vi "2086查询波浪仪参数.vi"(8 "error in (no error)":errorcluster, 10 "database":string="database1.mdb", 11 "table":string) -> (0 "error out":errorcluster, 1 "database溢出":bool, 2 "有数据":bool, 3 "data":string[][](array[string]), 4 "拆分数据":bool, 5 "columns":string[](array[string]))   [LabVIEW 2016, in "数据传输系统-05.lvlib"]
uses:
  <vilib>/Utility/sysdir.llb/System Directory Type.ctl
  <vilib>/addons/database/Connection.llb/DB Tools Open Connec (String).vi
  <vilib>/addons/database/Connection.llb/Conn Execute.vi
  <vilib>/addons/database/Recordset.llb/Rec Fetch Recordset Data (R).vi
  <vilib>/addons/database/Recordset.llb/Rec Destroy - Connection.vi
  <vilib>/addons/database/_DB Variant To Data/Database Variant To Data.xnode
  <vilib>/addons/database/NI_Database_API.lvlib
panel:
  out "连接的字符串":string
  out "结果字符串":string
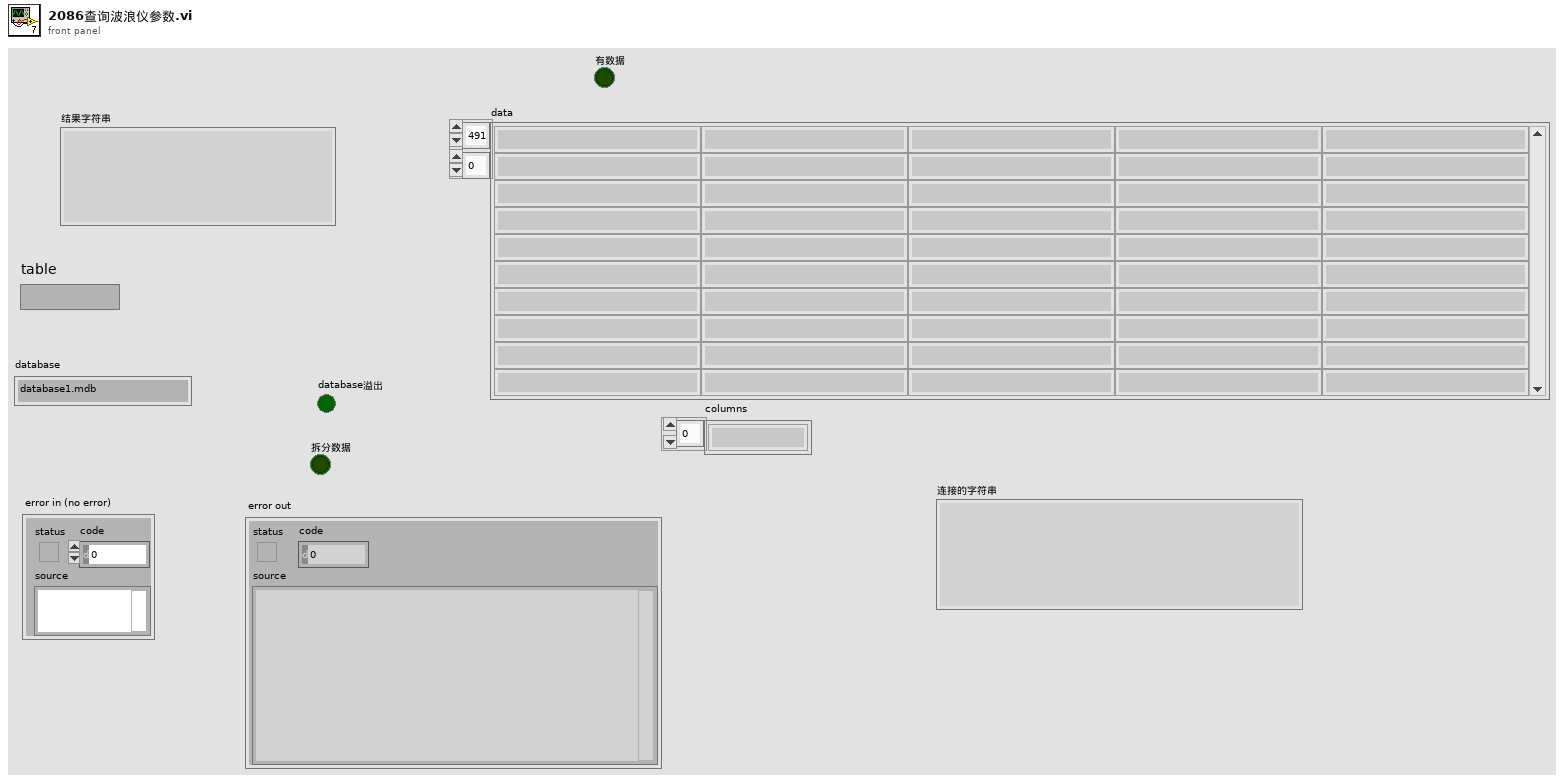
[diagram p1: front panel]
types:
  T1 = typedef "System Directory Type.ctl" = i32
  T2 = typedef "NI_Database_API.lvlib/Conn ObjectReference.ctl" = refnum<k1>
  T3 = typedef "NI_Database_API.lvlib/Rec ObjectReference.ctl" = refnum<k1>
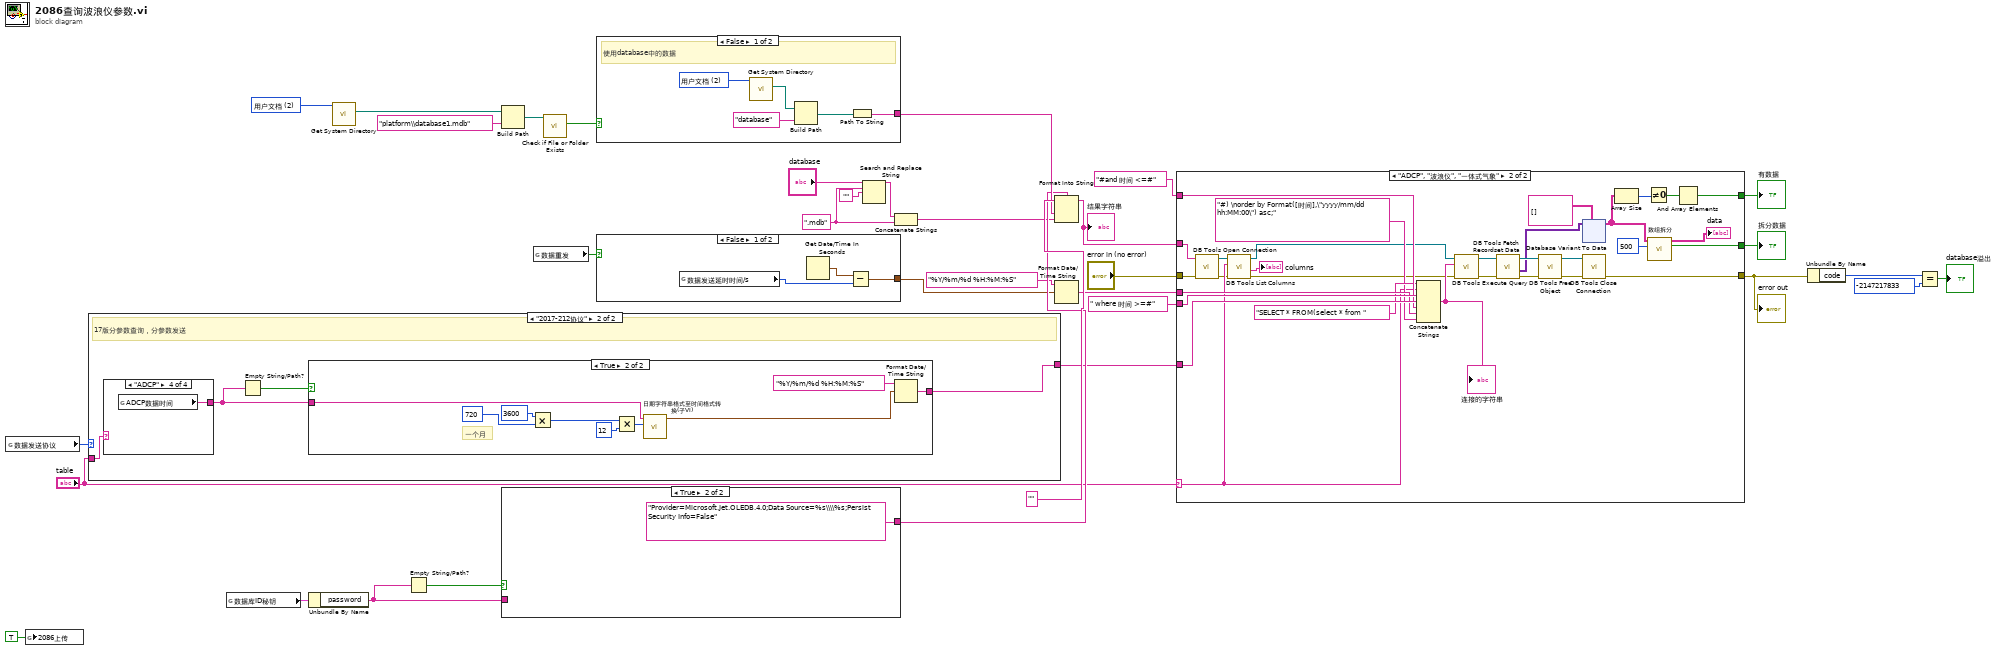
[diagram p0: block diagram]
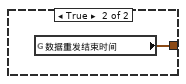
[diagram p2: hidden frame]
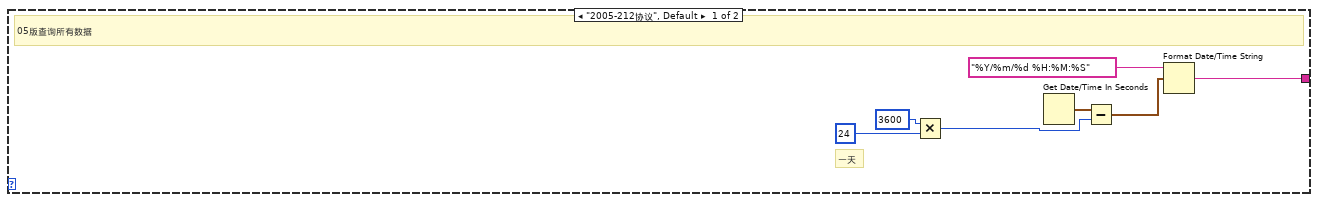
[diagram p3: hidden frame]
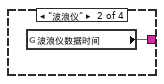
[diagram p5: hidden frame]
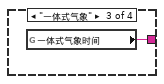
[diagram p6: hidden frame]
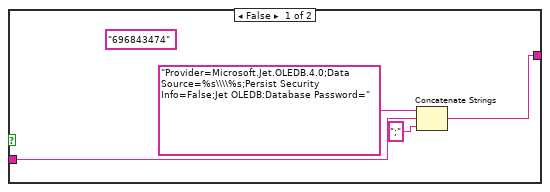
[diagram p9: hidden frame]
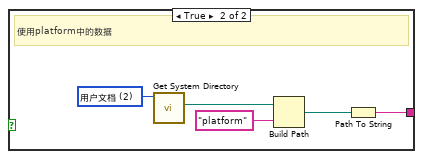
[diagram p10: hidden frame]
diagram:
  w19 = ".mdb" ("搜索字符串")
  w29 = T1 2 items=["用户目录"=0, "用户桌面"=1, "用户文档"=2, "用户应用程序数据"=3, "用户设置"=4, "用户临时目录"=5, "公共文档"=6, "公共应用程序数据"=7, "公共设置"=8, "公共缓存"=13, "系统核心库"=9, "系统安装库"=10, "应用程序文件"=11, "启动盘根目录"=12] ("system directory type")
  n1 = global read "断电保存全局.vi" "数据发送协议"() -> (w11:enum16{"2005-212协议", "2017-212协议"})
  n2 = global write "全局1.vi" "2086上传"(TRUE ("2086上传")) -> ()
  n3 = case shown="\"2017-212协议\"" w11 {
    tunnel: [w40 w45] -> w12
    tunnel: "table" -> [_ w42]
    frame "2005-212协议", Default {
      # "一天"
      # "05版查询所有数据"
      n4 = Multiply(x=3600, y=24) -> (x*y=w35:i32)
      n5 = Get Date/Time In Seconds() -> (seconds since 1Jan1904=w39:timestamp)
      n6 = Subtract(x=w39, y=w35) -> (x-y=w38:timestamp)
      n7 = Format Date/Time String(time format string (%c)="%Y/%m/%d %H:%M:%S" ("时间格式字符串(%c)"), seconds (now)=w38) -> (date/time string=w40:string)  [unwired: 1 in]
    }
    frame "2017-212协议" {
      # "17版分参数查询，分参数发送"
      n8 = case shown="\"ADCP\"" w42 {
        tunnel: [_ w46 w47 w48] -> w44
        frame "假", Default {
        }
        frame "波浪仪" {
          n9 = global read "全局 水样时间.vi" "波浪仪数据时间"() -> (w46:string)
        }
        frame "一体式气象" {
          n10 = global read "全局 水样时间.vi" "一体式气象时间"() -> (w47:string)
        }
        frame "ADCP" {
          n11 = global read "全局 水样时间.vi" "ADCP数据时间"() -> (w48:string)
        }
      }
      n12 = Empty String/Path?(string/path=w44) -> (empty?=w43:bool)
      n13 = case shown="True" w43 {
        tunnel: [w49 w55] -> w45
        tunnel: w44 -> [w49 w53]
        frame False {
        }
        frame True {
          # "一个月"
          n14 = Multiply(x=3600, y=720) -> (x*y=w52:i32)
          n15 = Multiply(x=w52, y=12) -> (x*y=w50:i32)
          n16 = call "日期字符串格式至时间格式转换(子VI).vi"("数值"=w50, "data[0]"=w53) -> ("time stamp"=w54:timestamp)  [unwired: 9 in]
          n17 = Format Date/Time String(time format string (%c)="%Y/%m/%d %H:%M:%S" ("时间格式字符串(%c)"), seconds (now)=w54) -> (date/time string=w55:string)  [unwired: 1 in]
        }
      }
    }
  }
  n18 = global read "外部交互全局.vi" "数据库ID秘钥"() -> (w22:cluster{"userID":string, "password":string})
  n19 = Unbundle By Name(w22) -> ("password"=w24:string)
  n20 = call <vilib>:"Get System Directory.vi"("system directory type"=w29) -> ("system directory"=w30:path)  [unwired: 10 in]
  n21 = Empty String/Path?(string/path=w24) -> (empty?=w3:bool)
  n22 = Build Path(base path=w30, name or relative path="platform\\database1.mdb" ("condition")) -> (appended path=w28:path)
  n23 = case shown="True" w3 {
    tunnel: [w60 "Provider=Microsoft.Jet.OLEDB.4.0;Data Source=%s\\\\%s;Persist Security Info=False" ("格式字符串")] -> w23
    tunnel: w24 -> [w59 _]
    frame False {
      (unwired) "696843474" ("格式字符串")
      n24 = Concatenate Strings("Provider=Microsoft.Jet.OLEDB.4.0;Data Source=%s\\\\%s;Persist Security Info=False;Jet OLEDB:Database Password=" ("格式字符串"), w59, ";" ("字符串")) -> (w60:string)
    }
    frame True {
    }
  }
  n25 = global read "断电保存全局.vi" "数据重发"() -> (w10:bool)
  n26 = call <vilib>:"Check if File or Folder Exists.vi"("path"=w28) -> ("file or folder exists?"=w26:bool)  [unwired: 8 in, 2 out]
  n27 = case shown="False" w26 {
    tunnel: [w64 w69] -> w25
    frame False {
      w67 = T1 2 items=["用户目录"=0, "用户桌面"=1, "用户文档"=2, "用户应用程序数据"=3, "用户设置"=4, "用户临时目录"=5, "公共文档"=6, "公共应用程序数据"=7, "公共设置"=8, "公共缓存"=13, "系统核心库"=9, "系统安装库"=10, "应用程序文件"=11, "启动盘根目录"=12] ("system directory type")
      # "使用database中的数据"
      n28 = call <vilib>:"Get System Directory.vi"("system directory type"=w67) -> ("system directory"=w66:path)  [unwired: 10 in]
      n29 = Build Path(base path=w66, name or relative path="database" ("condition")) -> (appended path=w68:path)
      n30 = Path To String(path=w68) -> (string=w64:string)
    }
    frame True {
      w73 = T1 2 items=["用户目录"=0, "用户桌面"=1, "用户文档"=2, "用户应用程序数据"=3, "用户设置"=4, "用户临时目录"=5, "公共文档"=6, "公共应用程序数据"=7, "公共设置"=8, "公共缓存"=13, "系统核心库"=9, "系统安装库"=10, "应用程序文件"=11, "启动盘根目录"=12] ("system directory type")
      # "使用platform中的数据"
      n31 = call <vilib>:"Get System Directory.vi"("system directory type"=w73) -> ("system directory"=w72:path)  [unwired: 10 in]
      n32 = Build Path(base path=w72, name or relative path="platform" ("condition")) -> (appended path=w70:path)
      n33 = Path To String(path=w70) -> (string=w69:string)
    }
  }
  n34 = case shown="False" w10 {
    tunnel: [w74 w77] -> w8
    frame False {
      n35 = global read "断电保存全局.vi" "数据发送延时时间/s"() -> (w75:i32)
      n36 = Get Date/Time In Seconds() -> (seconds since 1Jan1904=w76:timestamp)
      n37 = Subtract(x=w76, y=w75) -> (x-y=w74:timestamp)
    }
    frame True {
      n38 = global read "断电保存全局.vi" "数据重发结束时间"() -> (w77:timestamp)
    }
  }
  n39 = Search and Replace String(input string="database", search string=w19, replace string="") -> (result string=w20:string)  [unwired: 5 in, 3 out]
  n40 = Concatenate Strings(w20, w19) -> (w17:string)
  n41 = Format Into String(format string=w23, initial string="" ("初始字符串"), w25, w17) -> (resulting string=w13:string)  [unwired: 1 in, 1 out]
  "结果字符串" <- w13
  n42 = Format Date/Time String(time format string (%c)="%Y/%m/%d %H:%M:%S" ("时间格式字符串(%c)"), seconds (now)=w8) -> (date/time string=w7:string)  [unwired: 1 in]
  n43 = case shown="\"ADCP\", \"波浪仪\", \"一体式气象\"" "table" {
    selector: "table" -> [_ w83]
    tunnel: " where 时间 >=#" -> [_ w106]
    tunnel: w12 -> [_ w105]
    tunnel: "#and 时间 <=#" -> [_ w104]
    tunnel: w7 -> [_ w103]
    tunnel: "error in (no error)" -> [w78 w95]
    tunnel: [w78 w97] -> w14
    tunnel: w13 -> [_ w96]
    tunnel: [_ w88] -> w4
    tunnel: [_ w86] -> w2
    frame "假", Default {
    }
    frame "ADCP", "波浪仪", "一体式气象" {
      n44 = call-poly <vilib>:"DB Tools Open Connection.vi"("error in (no error)"=w95, "connection information"=w96) -> ("error out"=w82:errorcluster, "connection reference"=w85:T2)  [unwired: 6 in]
      n45 = call <vilib>:"DB Tools List Columns.vi"("error in (no error)"=w82, "table"=w83, "connection reference"=w85) -> ("error out"=w81:errorcluster, "columns"=→"columns":string[], "connection reference out"=w84:T2)  [unwired: 1 in, 1 out]
      n46 = Concatenate Strings("SELECT * FROM(select * from " ("连接的字符串"), w83, w106, w105, w104, w103, "#) \norder by Format([时间],\"yyyy/mm/dd hh:MM:00\") asc;" ("字符串")) -> (w91:string)
      "连接的字符串" <- w91
      n47 = call-poly <vilib>:"DB Tools Execute Query.vi"("error in (no error)"=w81, "SQL query"=w91, "connection reference"=w84) -> ("error out"=w109:errorcluster, "recordset reference"=w80:T3)  [unwired: 5 in]
      n48 = call-poly <vilib>:"DB Tools Fetch Recordset Data.vi"("error in (no error)"=w109, "recordset reference"=w80) -> ("error out"=w107:errorcluster, "recordset data"=w102:variant[][], "recordset reference out"=w108:T3)  [unwired: 3 in]
      n49 = call-poly <vilib>:"DB Tools Free Object.vi"("error in (no error)"=w107, "recordset reference"=w108) -> ("error out"=w98:errorcluster, "connection reference"=w99:T2)  [unwired: 8 in]
      n50 = xnode "Database Variant To Data"("database variant"=w102, "type"=string[][] []) -> ("data"=w87:string[][])  [unwired: 1 in, 1 out]
      n51 = call <vilib>:"DB Tools Close Connection.vi"("error in (no error)"=w98, "connection reference"=w99) -> ("error out"=w97:errorcluster)  [unwired: 5 in]
      n52 = Array Size(array=w87) -> (size(s)=w90:i32[])
      n53 = Not Equal To 0?(x=w90) -> (x != 0?=w89:bool[])
      n54 = call "数组拆分.vi"("拆分大小"=500, "输入数据"=w87) -> ("拆分数据"=w86:bool, "输出数组"=→"data":string[][])  [unwired: 8 in]
      n55 = And Array Elements(Boolean array=w89) -> (logical AND=w88:bool)
    }
  }
  "error out" <- w14
  "有数据" <- w4
  "拆分数据" <- w2
  n56 = Unbundle By Name(w14) -> ("code"=w34:i32)
  n57 = Equal?(x=w34, y=-2147217833 ("code")) -> (x = y?=→"database溢出":bool)
